vi "Handle Variable Header.vi"(8 "error in (no error)":errorcluster, 10 "Incoming Packets":u8[](array[numeric]) format="%08b", 11 "CONNACK in":refnum<class "CONNACK.lvclass">) -> (0 "error out":errorcluster, 1 "Variable Header Complete?":bool=TRUE, 2 "Remaining Packets":u8[](array[numeric]) format="%08b", 3 "CONNACK out":refnum<class "CONNACK.lvclass">)   [LabVIEW 2013, in "MQTT_Control_Packets.lvlib" / "CONNACK.lvclass"]
uses:
  CONNACK.lvclass
  ControlPacket/ControlPacket.lvclass/ControlPacket.ctl
  ControlPacket/ControlPacket.lvclass
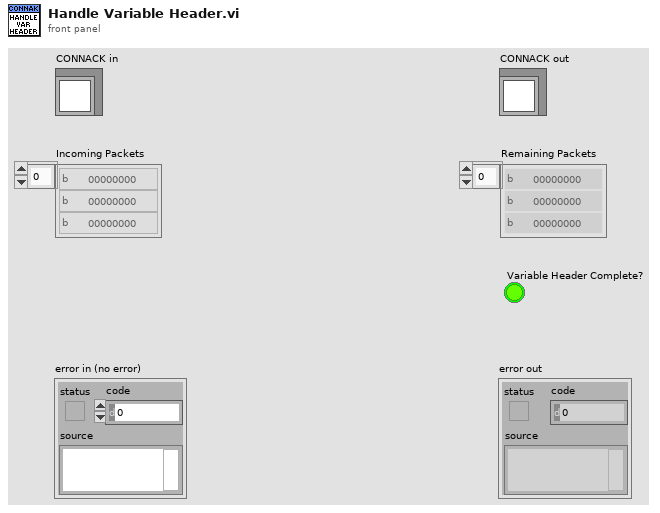
[diagram p1: front panel]
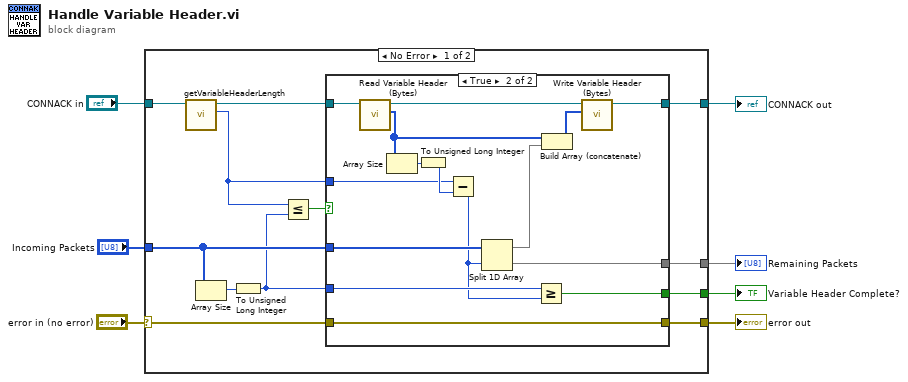
[diagram p0: block diagram]
diagram:
  n1 = case shown="No Error" "error in (no error)" {
    selector: "error in (no error)" -> [w8 w38]
    tunnel: "CONNACK in" -> [w18 w40]
    tunnel: "Incoming Packets" -> [w17 w39]
    tunnel: [w15 _] -> w2
    tunnel: [w14 w39] -> w3
    tunnel: [w13 w40] -> w4
    tunnel: [w9 w38] -> w1
    frame No Error {
      n2 = call-dynamic "getVariableHeaderLength.vi"("CONNACK in"=w18) -> ("VariableHeader size"=w11:u32, "CONNACK out"=w19:refnum<class "CONNACK.lvclass">)  [unwired: 8 in, 1 out]
      n3 = Array Size(array=w17) -> (size(s)=w16:i32)
      n4 = To Unsigned Long Integer(number=w16) -> (unsigned 32bit integer=w10:u32)
      n5 = Less Or Equal?(x=w11, y=w10) -> (x <= y?=w12:bool)
      n6 = case shown="True" w12 {
        tunnel: w19 -> [w20 w37]
        tunnel: w17 -> [w21 w30]
        tunnel: w10 -> [_ w29]
        tunnel: [_ w27] -> w15
        tunnel: [w21 w26] -> w14
        tunnel: [w20 w25] -> w13
        tunnel: w11 -> [_ w24]
        tunnel: [w22 w23] -> w9
        tunnel: w8 -> [w22 w23]
        frame False {
        }
        frame True {
          n7 = call "Read Variable Header (Bytes).vi"("ControlPacket in"=w37) -> ("Variable Header (Bytes)"=w34:u8[], "ControlPacket out"=w36:refnum<class "CONNACK.lvclass">)  [unwired: 9 in]
          n8 = Array Size(array=w34) -> (size(s)=w35:i32)
          n9 = To Unsigned Long Integer(number=w35) -> (unsigned 32bit integer=w31:u32)
          n10 = Subtract(x=w24, y=w31) -> (x-y=w28:u32)
          n11 = Split 1D Array(array=w30, index=w28) -> (first subarray=w33:u8[], second subarray=w26:u8[])
          n12 = Greater Or Equal?(x=w29, y=w28) -> (x >= y?=w27:bool)
          n13 = Build Array (concatenate)(w34, w33) -> (w32:u8[])
          n14 = call "Write Variable Header (Bytes).vi"("Variable Header (Bytes)"=w32, "ControlPacket in"=w36) -> ("ControlPacket out"=w25:refnum<class "CONNACK.lvclass">)  [unwired: 9 in]
        }
      }
    }
    frame Error {
    }
  }
  "error out" <- w1
  "CONNACK out" <- w4
  "Remaining Packets" <- w3
  "Variable Header Complete?" <- w2
